vi "init_main.vi"(8 "error in (no error)":errorcluster, 11 "VI in":refnum<vi>) -> (0 "error out":errorcluster)   [LabVIEW 2020]
uses:
  FGVs/FGVstates.ctl
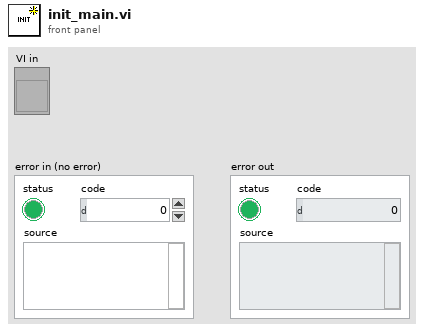
[diagram p1: front panel]
types:
  T1 = typedef "FGVstates.ctl" = enum16{"Init", "Set", "Get", "De-Init"}
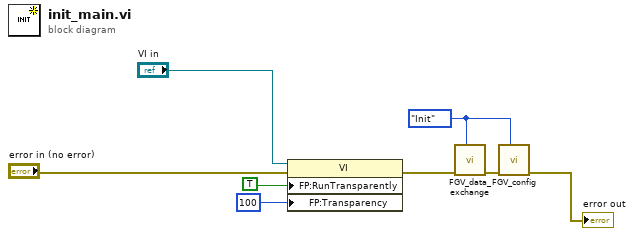
[diagram p0: block diagram]
diagram:
  w8 = FGVstates."Init" ("FGV states")
  n1 = property class="VI"(reference="VI in", error in="error in (no error)", "FP:RunTransparently"=TRUE ("Front Panel Window:Run VI Transparently"), "FP:Transparency"=u8 100 ("Front Panel Window:Transparency")) -> (error out=w1:errorcluster)  [unwired: 1 out]
  n2 = call "FGV_data_exchange.vi"("FGV states"=w8, "error in (no error)"=w1) -> ("error out"=w6:errorcluster)  [unwired: 8 in, 1 out]
  n3 = call "FGV_config.vi"("FGV states"=w8, "error in (no error)"=w6) -> ("error out"=→"error out":errorcluster)  [unwired: 8 in, 1 out]
